vi "Wiimote Set Output Report.vi"(8 "error in":errorcluster, 10 "pReportBuffer in":u8[](array[numeric]) format="%02x", 11 "hWiimoteHandle in":u32 format="%08x") -> (0 "error out":errorcluster, 3 "hWiimoteHandle out":u32 format="%08x")   [LabVIEW 2010]
uses:
  C:/Windows/System32/hid.dll
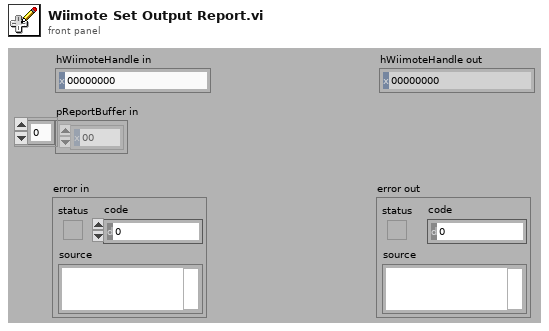
[diagram p1: front panel]
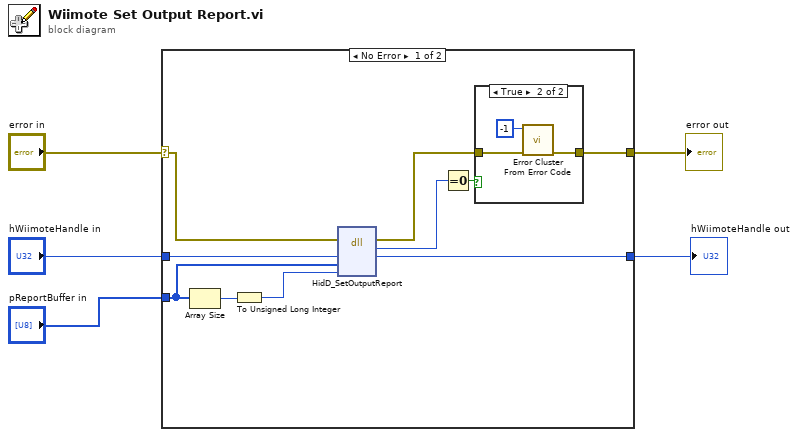
[diagram p0: block diagram]
diagram:
  n1 = case shown="No Error" "error in" {
    selector: "error in" -> [w11 w21]
    tunnel: [w10 w21] -> w4
    tunnel: "hWiimoteHandle in" -> [w15 w20]
    tunnel: "pReportBuffer in" -> [w14 _]
    tunnel: [w8 w20] -> w1
    frame No Error {
      n2 = Array Size(array=w14) -> (size(s)=w13:i32)
      n3 = To Unsigned Long Integer(number=w13) -> (unsigned 32bit integer=w12:u32)
      n4 = dll-call lib="C:/Windows/System32/hid.dll" fn="HidD_SetOutputReport"(error in=w11, "hWiimoteHandle"=w15, "pReportBuffer"=w14, "dwReportBufferLength"=w12) -> (error out=w9:errorcluster, "return type"=w6:u32, "hWiimoteHandle"=w8:u32)  [unwired: 4 in, 1 out]
      n5 = Equal To 0?(x=w6) -> (x = 0?=w7:bool)
      n6 = case shown="True" w7 {
        tunnel: w9 -> [w16 w19]
        tunnel: [w16 w18] -> w10
        frame False {
        }
        frame True {
          n7 = call <vilib>:"Error Cluster From Error Code.vi"("error in (no error)"=w19, "error code (0)"=-1) -> ("error out"=w18:errorcluster)  [unwired: 7 in]
        }
      }
    }
    frame Error {
    }
  }
  "error out" <- w4
  "hWiimoteHandle out" <- w1
